vi "kf_set_params.vi"(0 "KF in":T2={"A"=[], "B"=[], "H"=[], "Q"=[], "R"=[], "x"=[], "P"=[], "x lim"=[], "y lim"=[], "K"=[], "Converge count"=-1} {"K" format="%#_3g"; "y lim" format="%#_3g"; "x lim" format="%#_3g"; "P" format="%#_3g"; "H" format="%#_3g"; "x" format="%#_3g"; "Q" format="%#_3g"; "R" format="%#_3g"; "B" format="%#_3g"; "A" format="%#_3g"}, 1 "State limits":sgl[](array[numeric]), 2 "Innovation limits":sgl[](array[numeric]), 3 "Process noise":sgl[](array[numeric]), 4 "Initial input":T1, 5 "Measurement noise":sgl[](array[numeric]), 7 "A scale indices":cluster{"Row":i32, "Column":i32}[](array[cluster]), 9 "B scale indices":i32[](array[numeric]), 11 "Scale factor":sgl=1.0, 13 "Converge count":i32=-1) -> (14 "KF out":T2={"A"=[], "B"=[], "H"=[], "Q"=[], "R"=[], "x"=[], "P"=[], "x lim"=[], "y lim"=[], "K"=[], "Converge count"=-1} {"K" format="%#_3g"; "y lim" format="%#_3g"; "x lim" format="%#_3g"; "P" format="%#_3g"; "H" format="%#_3g"; "x" format="%#_3g"; "Q" format="%#_3g"; "R" format="%#_3g"; "B" format="%#_3g"; "A" format="%#_3g"})   [LabVIEW 2014]
uses:
  kalman_filter.ctl
  <vilib>/Analysis/Matrix/Datatypes/RealMatrix.ctl
  <vilib>/Analysis/baseanly.llb/Real A x B.vi
  <vilib>/Analysis/NI_AALBase.lvlib
  <vilib>/Analysis/Matrix/NI_Matrix.lvlib
panel:
  # "This VI provides a convenient way to set the KF fields that are likely to want to be run-time tunable.  If an argument is empty (unsupplied), then the existing values are not changed."
  # "The diagonals of Q and R are set to the square of these values.  Extra values are ignored.  Q data is scaled after squaring (see \"Scale factor\").  R is also used to initialize P, if has not been initialized yet (is all zero.)"
  # "Copy into the \"x lim\" and \"y lim\" fields, preserving the existing\nmatrix size.  \"y lim\" is scaled (see \"Scale factor\".)"
  # "Scale some elements of the system definition matrices.  Useful to parameterize by sample interval."
  # "If non-empty, sets the state according to the input.  \n    x = H' * z\nThis evades problems with innovation limits when the filter is initializing.   If P is uninitialized (0), we will also set P to H'RH, setting the state covariance according to the measurement noise, so the effect is the same as making a first measurement.   If you don't supply this on the first call, then you have effectively used zero as the initial measurement."
  # "Set to positive value to indicate number of cycles until steady state.  Steady state update is faster."
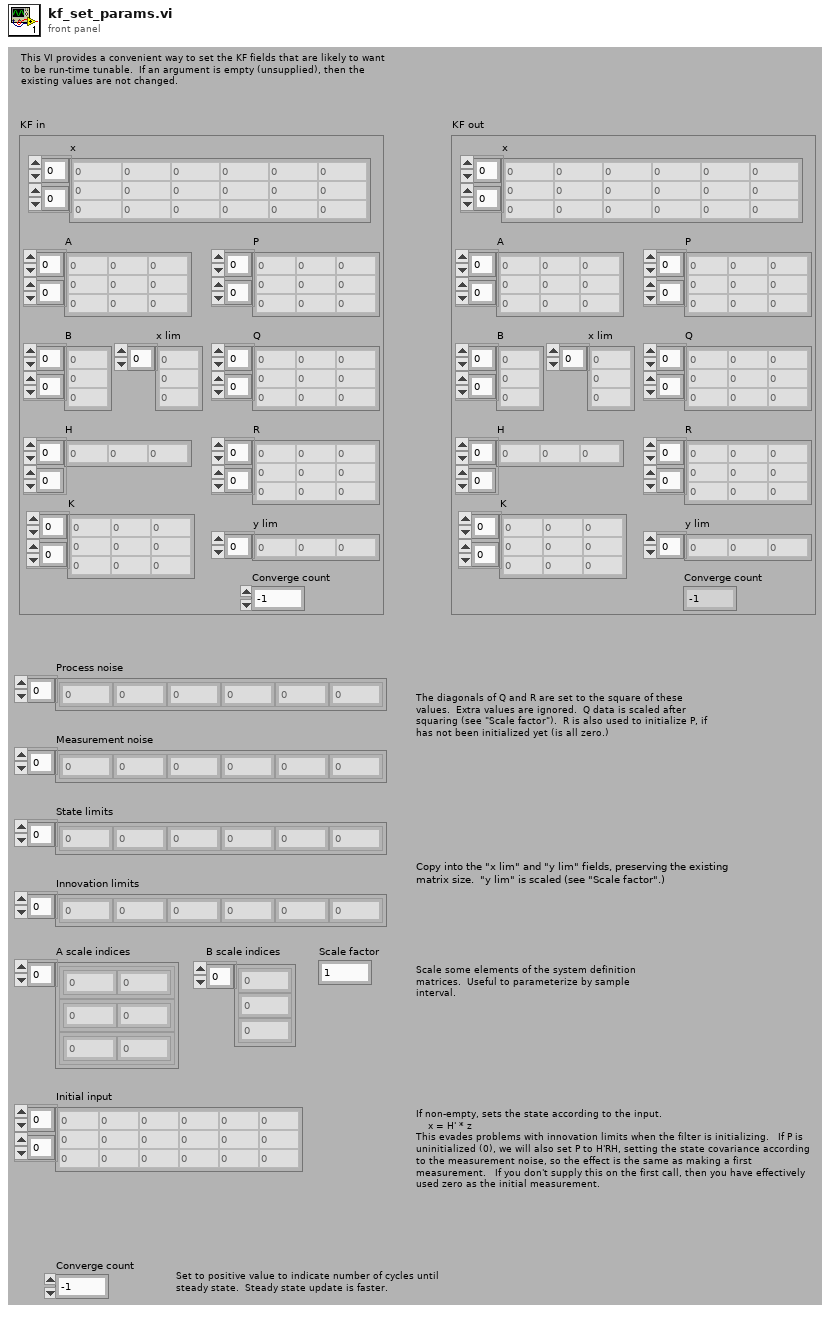
[diagram p1: front panel]
types:
  T1 = typedef "NI_Matrix.lvlib/RealMatrix.ctl" = dbl[][]
  T2 = typedef "kalman_filter.ctl" = cluster{"A":T1, "B":T1, "H":T1, "Q":T1, "R":T1, "x":T1, "P":T1, "x lim":dbl[], "y lim":dbl[], "K":T1, "Converge count":i32}
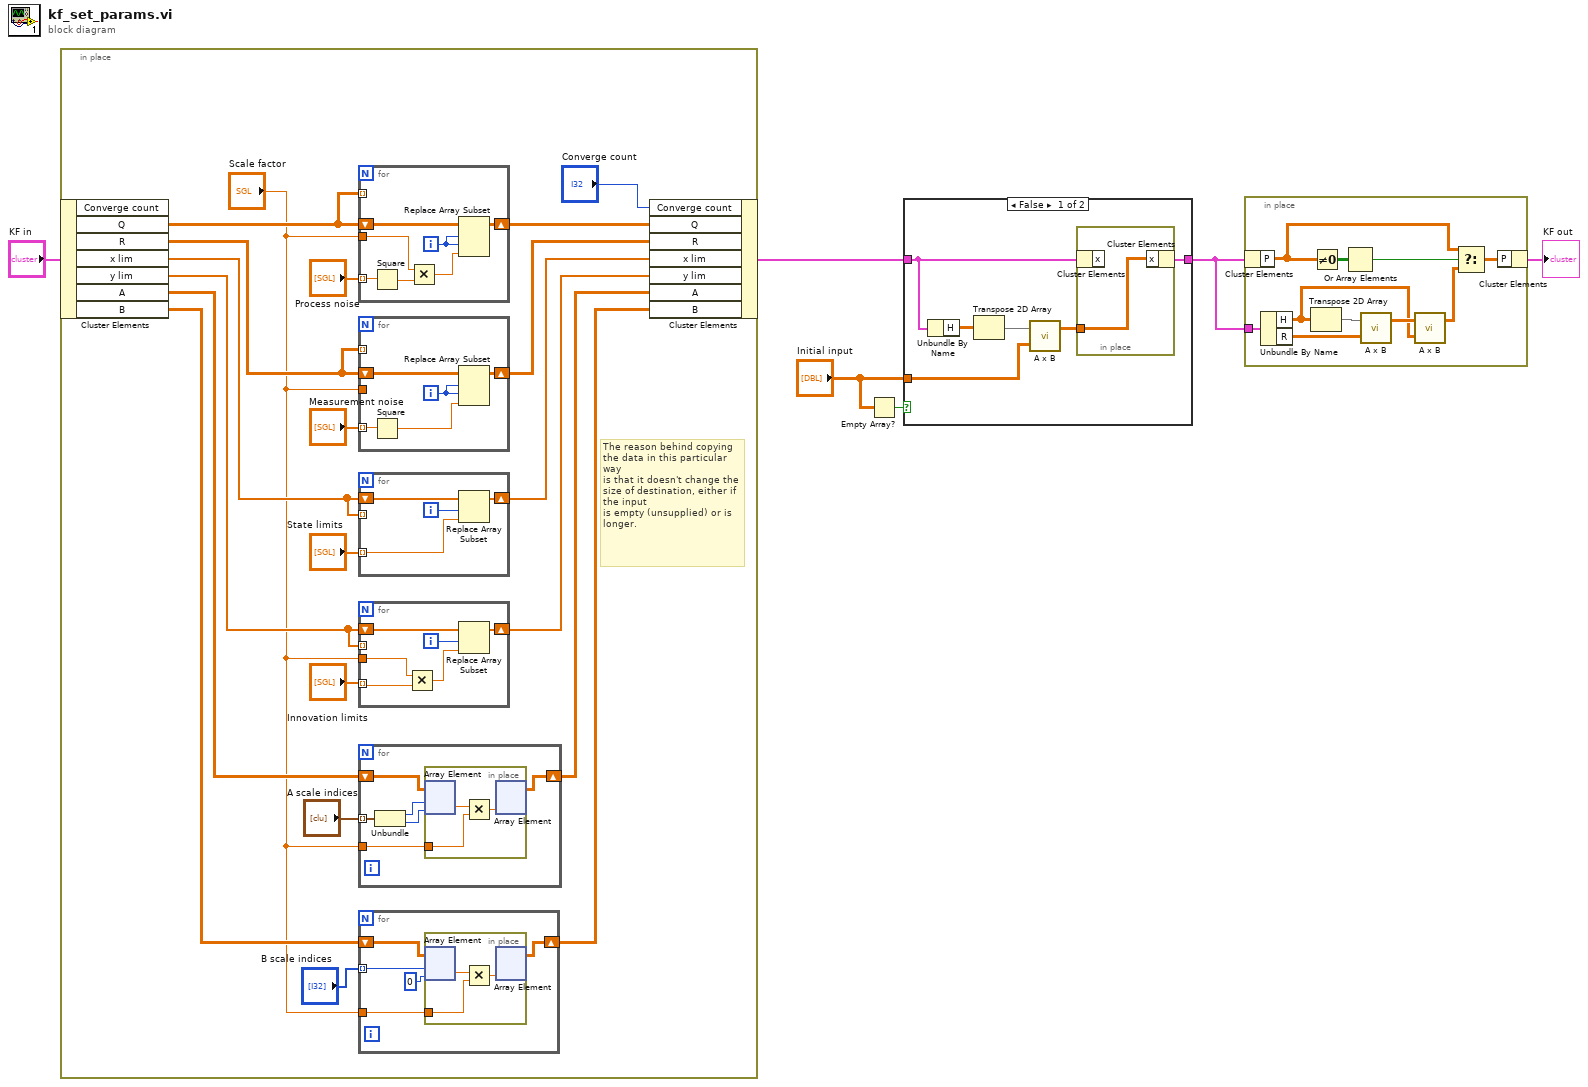
[diagram p0: block diagram]
diagram:
  n1 = in-place {
    # "The reason behind copying the data in this particular way\nis that it doesn't change the size of destination, either if the input\nis empty (unsupplied) or is longer."
    n2 = in-place-cluster #1("KF in") -> ("Q"=w26:T1, "R"=w22:T1, "x lim"=w16:dbl[], "y lim"=w15:dbl[], "A"=w13:T1, "B"=w10:T1)  [unwired: 1 out]
    n3 = for {
      tunnel: w26 -> [_] mode=indexing
      tunnel: "Process noise" -> [w62] mode=indexing
      shift-right: [w63] -> w24
      shift-left: w26 -> [w65]
      tunnel: "Scale factor" -> [w60]
      i -> [w64]
      n4 = Square(x=w62) -> (x^2=w61:sgl)
      n5 = Multiply(x=w60, y=w61) -> (x*y=w59:sgl)
      n6 = Replace Array Subset(array=w65, new element=w59, index (row)=w64, index (col)=w64) -> (w63:T1)
    }
    n7 = for {
      tunnel: "Measurement noise" -> [w55] mode=indexing
      tunnel: w22 -> [_] mode=indexing
      shift-right: [w56] -> w21
      shift-left: w22 -> [w58]
      tunnel: "Scale factor" -> [_]
      i -> [w57]
      n8 = Square(x=w55) -> (x^2=w54:sgl)
      n9 = Replace Array Subset(array=w58, new element=w54, index (row)=w57, index (col)=w57) -> (w56:T1)
    }
    n10 = for {
      tunnel: "State limits" -> [w50] mode=indexing
      shift-right: [w51] -> w19
      shift-left: w16 -> [w53]
      tunnel: w16 -> [_] mode=indexing
      i -> [w52]
      n11 = Replace Array Subset(array=w53, new element=w50, index=w52) -> (w51:dbl[])
    }
    n12 = for {
      tunnel: "Innovation limits" -> [w46] mode=indexing
      shift-right: [w47] -> w18
      shift-left: w15 -> [w49]
      tunnel: w15 -> [_] mode=indexing
      tunnel: "Scale factor" -> [w45]
      i -> [w48]
      n13 = Multiply(x=w45, y=w46) -> (x*y=w44:sgl)
      n14 = Replace Array Subset(array=w49, new element=w44, index=w48) -> (w47:dbl[])
    }
    n15 = for {
      tunnel: "A scale indices" -> [w39] mode=indexing
      tunnel: "Scale factor" -> [w36]
      shift-right: [w35] -> w12
      shift-left: w13 -> [w40]
      n16 = Unbundle(w39) -> ("Row"=w38:i32, "Column"=w37:i32)
      n17 = in-place {
        in-place-border: w36 -> [w41]
        n18 = in-place-array #2(w40, w38, w37) -> (w43:dbl)
        n19 = Multiply(x=w43, y=w41) -> (x*y=w42:dbl)
        n20 = in-place-array #2(w42) -> (w35:T1)  [unwired: 2 out]
      }
    }
    n21 = for {
      tunnel: "Scale factor" -> [w30]
      tunnel: "B scale indices" -> [w28] mode=indexing
      shift-right: [w29] -> w9
      shift-left: w10 -> [w31]
      n22 = in-place {
        in-place-border: w30 -> [w32]
        n23 = in-place-array #3(w31, w28, 0) -> (w34:dbl)
        n24 = Multiply(x=w34, y=w32) -> (x*y=w33:dbl)
        n25 = in-place-array #3(w33) -> (w29:T1)  [unwired: 2 out]
      }
    }
    n26 = in-place-cluster #1("Converge count"="Converge count", "Q"=w24, "R"=w21, "x lim"=w19, "y lim"=w18, "A"=w12, "B"=w9) -> (w3:T2)
  }
  n27 = Empty Array?(array="Initial input") -> (empty?=w4:bool)
  n28 = case shown="False" w4 {
    tunnel: "Initial input" -> [w70 _]
    tunnel: w3 -> [w71 w73]
    tunnel: [w67 w73] -> w2
    frame False {
      n29 = Unbundle By Name(w71) -> ("H"=w66:T1)
      n30 = Transpose 2D Array(2D array=w66) -> (transposed array=w68:T1)
      n31 = call-poly <vilib>:"A x B.vi"("B"=w70, "A"=w68) -> ("A x B"=w69:T1)  [unwired: 1 out]
      n32 = in-place {
        in-place-border: w69 -> [w72]
        n33 = in-place-cluster #4(w71) -> ()  [unwired: 1 out]
        n34 = in-place-cluster #4("x"=w72) -> (w67:T2)
      }
    }
    frame True {
    }
  }
  n35 = in-place {
    in-place-border: w2 -> [w79]
    n36 = in-place-cluster #5(w2) -> ("P"=w83:T1)
    n37 = Unbundle By Name(w79) -> ("H"=w75:T1, "R"=w77:T1)
    n38 = Transpose 2D Array(2D array=w75) -> (transposed array=w78:T1)
    n39 = Not Equal To 0?(x=w83) -> (x != 0?=w82:bool[][])
    n40 = Or Array Elements(Boolean array=w82) -> (logical OR=w81:bool)
    n41 = call-poly <vilib>:"A x B.vi"("B"=w77, "A"=w78) -> ("A x B"=w76:T1)  [unwired: 1 out]
    n42 = call-poly <vilib>:"A x B.vi"("B"=w75, "A"=w76) -> ("A x B"=w74:T1)  [unwired: 1 out]
    n43 = Select(t=w83, s=w81, f=w74) -> (s? t:f=w80:T1)
    n44 = in-place-cluster #5("P"=w80) -> (→"KF out":T2)
  }
